vi "UTM_trans (SubVI).vi"(4 "Long_Deg":dbl, 5 "long":dbl format="%#_13g", 6 "lat":dbl format="%#_12g", 7 "East?West?":bool=TRUE, 8 "Lat_Deg":dbl) -> (0 "Display_Long":dbl, 1 "Display_Lat":dbl, 2 "UTM_Y(Northing)":dbl format="%#_15g", 3 "UTM_X(Easting)":dbl format="%#_16g")   [LabVIEW 2024]
panel:
  # "NMEA Format"
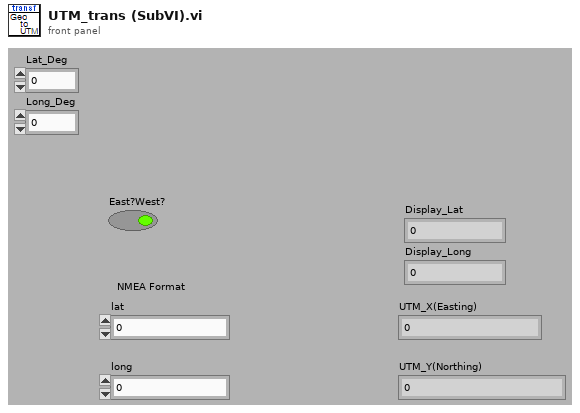
[diagram p1: front panel]
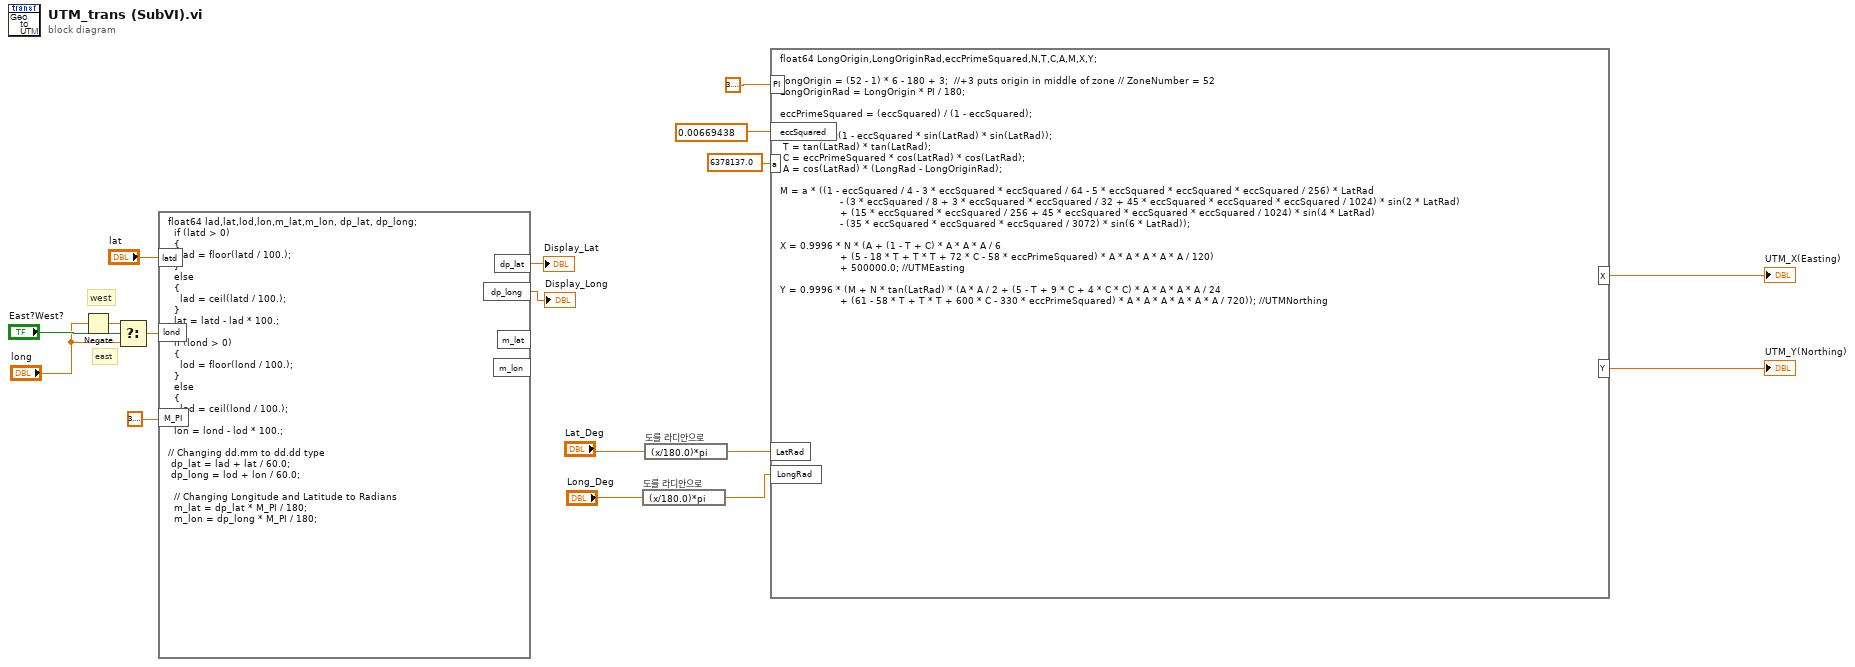
[diagram p0: block diagram]
diagram:
  # "east"
  # "west"
  n1 = Negate(x="long") -> (-x=w9:dbl)
  n2 = Select(t=w9, s="East?West?", f="long") -> (s? t:f=w7:dbl)
  n3 = formula code="float64 lad,lat,lod,lon,m_lat,m_lon, dp_lat, dp_long;\n  if (latd > 0)\n  {\n    lad = floor(latd / 100.);\n  }\n  else\n  {\n    lad = ceil(latd / 100.);\n  }\n  lat = latd - lad * 100.;\n\n  if (lond > 0)\n  {\n    lod = floor(lond / 100.);\n  }\n  else\n  {\n    lod = ceil(lond / 100.);\n  }\n  lon = lond - lod * 100.;\n\n// Changing dd.mm to dd.dd type\n dp_lat = lad + lat / 60.0;\n dp_long = lod + lon / 60.0;\n\n  // Changing Longitude and Latitude to Radians\n  m_lat = dp_lat * M_PI / 180;\n  m_lon = dp_long * M_PI / 180;"("latd"="lat", "lond"=w7, "M_PI"=3.141592653589793) -> ("dp_lat"=→"Display_Lat":dbl, "dp_long"=→"Display_Long":dbl)  [unwired: 2 out]
  n4 = expression code="(x/180.0)*pi" "도를 라디안으로"("Long_Deg") -> (w1:dbl)
  n5 = expression code="(x/180.0)*pi" "도를 라디안으로"("Lat_Deg") -> (w2:dbl)
  n6 = formula code="float64 LongOrigin,LongOriginRad,eccPrimeSquared,N,T,C,A,M,X,Y;\n\nLongOrigin = (52 - 1) * 6 - 180 + 3;  //+3 puts origin in middle of zone // ZoneNumber = 52\nLongOriginRad = LongOrigin * PI / 180;\n\neccPrimeSquared = (eccSquared) / (1 - eccSquared);\n\n N = a / sqrt(1 - eccSquared * sin(LatRad) * sin(LatRad));\n T = tan(LatRad) * tan(LatRad);\n C = eccPrimeSquared * cos(LatRad) * cos(LatRad);\n A = cos(LatRad) * (LongRad - LongOriginRad);\n\nM = a * ((1 - eccSquared / 4 - 3 * eccSquared * eccSquared / 64 - 5 * eccSquared * eccSquared * eccSquared / 256) * LatRad\n                    - (3 * eccSquared / 8 + 3 * eccSquared * eccSquared / 32 + 45 * eccSquared * eccSquared * eccSquared / 1024) * sin(2 * LatRad)\n                    + (15 * eccSquared * eccSquared / 256 + 45 * eccSquared * eccSquared * eccSquared / 1024) * sin(4 * LatRad)\n                    - (35 * eccSquared * eccSquared * eccSquared / 3072) * sin(6 * LatRad));\n\nX = 0.9996 * N * (A + (1 - T + C) * A * A * A / 6\n                    + (5 - 18 * T + T * T + 72 * C - 58 * eccPrimeSquared) * A * A * A * A * A / 120)\n                    + 500000.0; //UTMEasting\n\nY = 0.9996 * (M + N * tan(LatRad) * (A * A / 2 + (5 - T + 9 * C + 4 * C * C) * A * A * A * A / 24\n                    + (61 - 58 * T + T * T + 600 * C - 330 * eccPrimeSquared) * A * A * A * A * A * A / 720)); //UTMNorthing"("LatRad"=w2, "LongRad"=w1, "PI"=3.141592653589793, "eccSquared"=0.00669438, "a"=6378137.0) -> ("X"=→"UTM_X(Easting)":dbl, "Y"=→"UTM_Y(Northing)":dbl)
